vi "DebugCompile.vi"(8 "error out 2":errorcluster, 11 "VS References in":T1 {"Refs"."Command Chanels" format="%.0x"; "Refs"."Status" format="%.0x"; "Refs"."DTCs" format="%.0x"; "Refs"."Number of DTCs" format="%.0x"; "Refs"."Write Data"."Refs"."Data Reference" format="%.0x"; "Refs"."Read Data" format="%.0x"; "Properties"."Writes"."Signals"."Byte Order" items=["Little Endian", "Big Endian"]; "Properties"."Writes"."Signals"."Data Type" items=["Signed", "Unsigned", "IEEE Float"]; "Properties"."CAN"."Fill Byte" format="%.0x"; "Properties"."CAN"."VW TP Channel ID" format="%.0x"; "Properties"."CAN"."Receive UUDT ID" format="%.0x"; "Properties"."CAN"."Receive Extension" format="%.0x"; "Properties"."CAN"."Transmit Extension" format="%.0x"; "Properties"."CAN"."Receive ID" format="%.0x"; "Properties"."CAN"."Transmit ID" format="%.0x"; "Properties"."Reads"."Signals"."Byte Order" items=["Little Endian", "Big Endian"]; "Properties"."Reads"."Signals"."Data Type" items=["Signed", "Unsigned", "IEEE Float"]}) -> ()   [LabVIEW 2015, in "Diagnostics Addon System Explorer.lvlib"]
uses:
  Diagnostics Addon System Explorer.lvlib
  Shared/Types/Compiled.Settings.ctl
  Shared/Types/Section Properties.ctl
  Shared/Types/CAN Configuration.ctl
  Shared/Types/CAN Interface.ctl
  Shared/Types/Diagnostic Protocols.ctl
  Shared/Types/Transport Protocols.ctl
  Shared/Types/Security.ctl
  Shared/Types/FPGA Bitfile Settings.ctl
  Shared/Types/Common Frame Parameters.ctl
  Shared/Types/MessageType Selector.ctl
  Shared/Types/Signal Parameters.ctl
  Shared/Types/DPID Parameters.ctl
  Shared/Types/DPID Periodic Rate.ctl
  <vilib>/Automotive Diagnostic Command Set/Diagnostic Protocols.llb/DTC Descriptor.ctl
  Shared/Types/Compiled.Refs.ctl
  <vilib>/NI Veristand/Custom Device API/Data Reference.ctl
  <vilib>/NI Veristand/Custom Device API/Block Data Reference.ctl
  Shared/Diagnostics Addon Shared.lvlib
  <vilib>/NI Veristand/Custom Device API/Custom Device API.lvlib
panel:
  in  "OK Button":bool
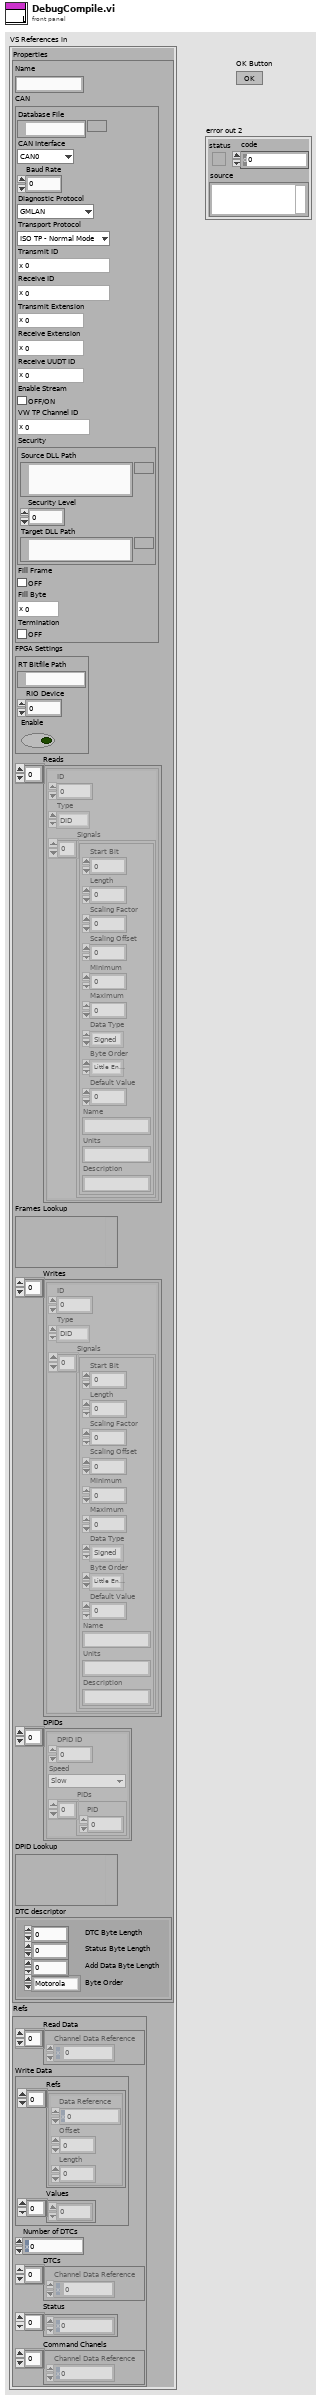
[diagram p1: front panel]
types:
  T1 = typedef "Diagnostics Addon Shared.lvlib/Compiled.Settings.ctl" = cluster{"Properties":T2, "Refs":T15}
  T2 = typedef "Diagnostics Addon Shared.lvlib/Section Properties.ctl" = cluster{"Name":string, "CAN":T3, "FPGA Settings":T8, "Reads":T9[], "Frames Lookup":variant, "Writes":T9[], "DPIDs":T12[], "DPID Lookup":variant, "DTC descriptor":T14}
  T3 = typedef "Diagnostics Addon Shared.lvlib/CAN Configuration.ctl" = cluster{"Database File":path, "CAN Interface":T4, "Baud Rate":u32, "Diagnostic Protocol":T5, "Transport Protocol":T6, "Transmit ID":u32, "Receive ID":u32, "Transmit Extension":u8, "Receive Extension":u8, "Receive UUDT ID":u32, "Enable Stream":bool, "VW TP Channel ID":u32, "Security":T7, "Fill Frame":bool, "Fill Byte":u8, "Termination":bool}
  T4 = typedef "Diagnostics Addon Shared.lvlib/CAN Interface.ctl" = enum16{"CAN0", "CAN1", "CAN2", "CAN3", "CAN4", "CAN5", "CAN6", "CAN7", "CAN8", "CAN9", "CAN10", "CAN11", "CAN12", "CAN13", "CAN14", "CAN15", "CAN16", "CAN17", "CAN18", "CAN19", "CAN20", "CAN21", "CAN22", "CAN23", "CAN24", "CAN25", "CAN26", "CAN27", "CAN28", "CAN29", "CAN30", "CAN31", "CAN32", "CAN33", "CAN34", "CAN35", "CAN36", "CAN37", "CAN38", "CAN39", "CAN40", "CAN41", "CAN42", "CAN43", "CAN44", "CAN45", "CAN46", "CAN47", "CAN48", "CAN49", "CAN50", "CAN51", "CAN52", "CAN53", "CAN54", "CAN55", "CAN56", "CAN57", "CAN58", "CAN59", "CAN60", "CAN61", "CAN62", "CAN63", "CAN 256 (Virtual)", "CAN 257 (Virtual)"}
  T5 = typedef "Diagnostics Addon Shared.lvlib/Diagnostic Protocols.ctl" = enum16{"GMLAN", "KWP-2000", "UDS"}
  T6 = typedef "Diagnostics Addon Shared.lvlib/Transport Protocols.ctl" = enum16{"ISO TP - Normal Mode", "ISO TP - Mixed Mode", "VW TP 2.0", "Diagnostics on IP"}
  T7 = typedef "Diagnostics Addon Shared.lvlib/Security.ctl" = cluster{"Source DLL Path":path, "Security Level":u8, "Target DLL Path":path}
  T8 = typedef "Diagnostics Addon Shared.lvlib/FPGA Bitfile Settings.ctl" = cluster{"RT Bitfile Path":path, "RIO Device":u16, "Enable":bool}
  T9 = typedef "Diagnostics Addon Shared.lvlib/Common Frame Parameters.ctl" = cluster{"ID":u32, "Type":T10, "Signals":T11[]}
  T10 = typedef "Diagnostics Addon Shared.lvlib/MessageType Selector.ctl" = enum16{"DID", "PID", "CPID", "Write Memory", "Read Memory", "DTC Control", "IO Cmd", "IO Resp", "Routine Start Cmd", "Routine Start Resp", "Routine Status Cmd", "Routine Status Resp", "Routine Stop Cmd", "Routine Stop Resp"}
  T11 = typedef "Diagnostics Addon Shared.lvlib/Signal Parameters.ctl" = cluster{"Start Bit":u8, "Length":u8, "Scaling Factor":dbl, "Scaling Offset":dbl, "Minimum":dbl, "Maximum":dbl, "Data Type":u32, "Byte Order":u32, "Default Value":dbl, "Name":string, "Units":string, "Description":string}
  T12 = typedef "Diagnostics Addon Shared.lvlib/DPID Parameters.ctl" = cluster{"DPID ID":u8, "Speed":T13, "PIDs":u16[]}
  T13 = typedef "Diagnostics Addon Shared.lvlib/DPID Periodic Rate.ctl" = enum16{"Slow", "Medium", "Fast"}
  T14 = typedef "Diagnostics Addon Shared.lvlib/DTC Descriptor.ctl" = cluster{"DTC Byte Length":i32, "Status Byte Length":i32, "Add Data Byte Length":i32, "Byte Order":enum16{"Motorola", "Intel"}}
  T15 = typedef "Diagnostics Addon Shared.lvlib/Compiled.Refs.ctl" = cluster{"Read Data":T16[], "Write Data":cluster{"Refs":T17[], "Values":dbl[]}, "Number of DTCs":T16, "DTCs":T16[], "Status":T16[], "Command Chanels":T16[]}
  T16 = typedef "Custom Device API.lvlib/Data Reference.ctl" = i32
  T17 = typedef "Custom Device API.lvlib/Block Data Reference.ctl" = cluster{"Data Reference":T16, "Offset":u64, "Length":u64}
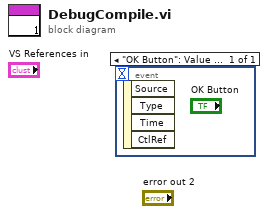
[diagram p0: block diagram]
diagram:
  n1 = event shown="[0] \"OK Button\": Value Change" {
    selector: _ -> [_]
    dyn-events: _ -> [_]
    timeout: _ -> [_]
    event "OK Button": Value Change {
      n2 = event-data() -> ()  [unwired: 1 in, 4 out]
    }
  }
